vi "GV mem address.vi"() -> ()   [LabVIEW 2017]
panel:
  out "Mem address":u16
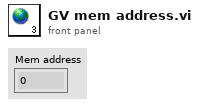
[diagram p1: front panel]
diagram:
